vi "getVIOutputs.vi"(8 "error in (no error)":errorcluster, 11 "Panel in":refnum<class "Panel.lvclass">) -> (0 "error out":errorcluster, 2 "UI.lvclass":refnum<class "UI.lvclass">, 3 "Panel out":refnum<class "Panel.lvclass">)   [LabVIEW 2019, in "Panel.lvclass"]
uses:
  Panel.lvclass
  User Interface/UI.lvclass
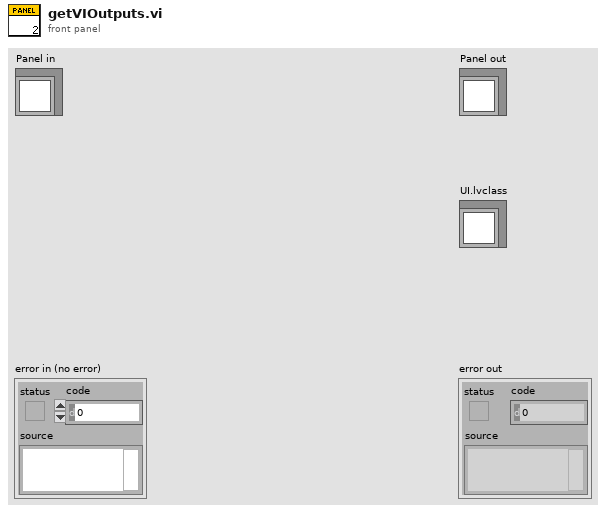
[diagram p1: front panel]
types:
  T1 = enum16{"Open Reference", "Launch VI", "Get VI Outputs"}
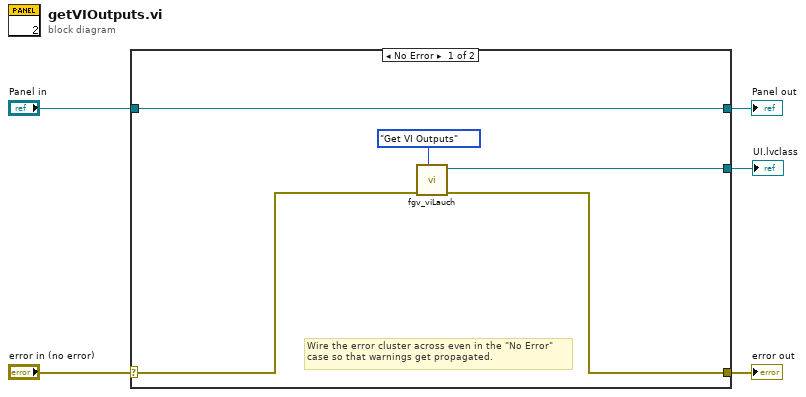
[diagram p0: block diagram]
diagram:
  n1 = case shown="No Error" "error in (no error)" {
    selector: "error in (no error)" -> [w8 w12]
    tunnel: [w7 w12] -> w4
    tunnel: [w10 w11] -> w2
    tunnel: "Panel in" -> [w10 w11]
    tunnel: [w9 _] -> w1
    frame No Error {
      # "Wire the error cluster across even in the \"No Error\"\ncase so that warnings get propagated."
      n2 = call "fgv_viLauch.vi"("Option"=T1."Get VI Outputs", "Error In"=w8) -> ("Error Out"=w7:errorcluster, "UI out"=w9:refnum<class "UI.lvclass">)  [unwired: 7 in, 1 out]
    }
    frame Error {
    }
  }
  "error out" <- w4
  "Panel out" <- w2
  "UI.lvclass" <- w1
